vi "OpenLEDStrip.vi"(0 "Digital Module (Module 1)":T2, 1 "Max Duty Cycle (1)":sgl=1.0, 5 "DIO Channel Red":T1, 7 "DIO Channel Green":T1, 9 "DIO Channel Blue":T1, 11 "error in (no error)":errorcluster, 12 "PWM Rate (Hz)":sgl=1000.0) -> (4 "LEDStripRef":T3={"PWM Rate (Hz)"=1000.0, "Max Duty Cycle"=1000.0, "DigitalOutputRed"={"Digital Module"=enum."Digital Module 1", "DIO Channel"=enum."DIO 1", "DevStatus"={"status"=FALSE, "code"=0, "source"=""}}, "DigitalOutputGreen"={"Digital Module"=enum."Digital Module 1", "DIO Channel"=enum."DIO 1", "DevStatus"={"status"=FALSE, "code"=0, "source"=""}}, "DigitalOutputBlue"={"Digital Module"=enum."Digital Module 1", "DIO Channel"=enum."DIO 1", "DevStatus"={"status"=FALSE, "code"=0, "source"=""}}, "DevStatus"={"status"=FALSE, "code"=0, "source"=""}}, 15 "error out":errorcluster)   [LabVIEW 2013]
uses:
  LEDStripRef.ctl
  <vilib>/Rock Robotics/WPI/DigitalOutput/WPI_DigitalOutputDevRef.ctl
  <vilib>/Rock Robotics/SystemInterfaces/Typedef/FPGA_TypedefDigitalModule.ctl
  <vilib>/Rock Robotics/SystemInterfaces/DIO/FPGA_DIOChannel.ctl
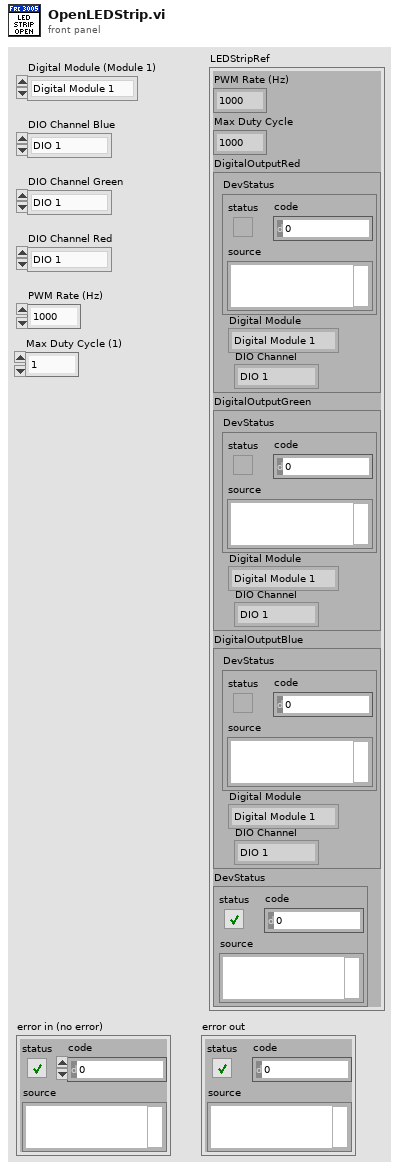
[diagram p1: front panel]
types:
  T1 = typedef "FPGA_DIOChannel.ctl" = enum8{"DIO 1", "DIO 2", "DIO 3", "DIO 4", "DIO 5", "DIO 6", "DIO 7", "DIO 8", "DIO 9", "DIO 10", "DIO 11", "DIO 12", "DIO 13", "DIO 14", "Invalid"}
  T2 = typedef "FPGA_TypedefDigitalModule.ctl" = enum16{"Digital Module 1", "Digital Module 2"}
  T3 = typedef "LEDStripRef.ctl" = cluster{"PWM Rate (Hz)":sgl, "Max Duty Cycle":sgl, "DigitalOutputRed":T4, "DigitalOutputGreen":T4, "DigitalOutputBlue":T4, "DevStatus":errorcluster}
  T4 = typedef "WPI_DigitalOutputDevRef.ctl" = cluster{"Digital Module":T2, "DIO Channel":T1, "DevStatus":errorcluster}
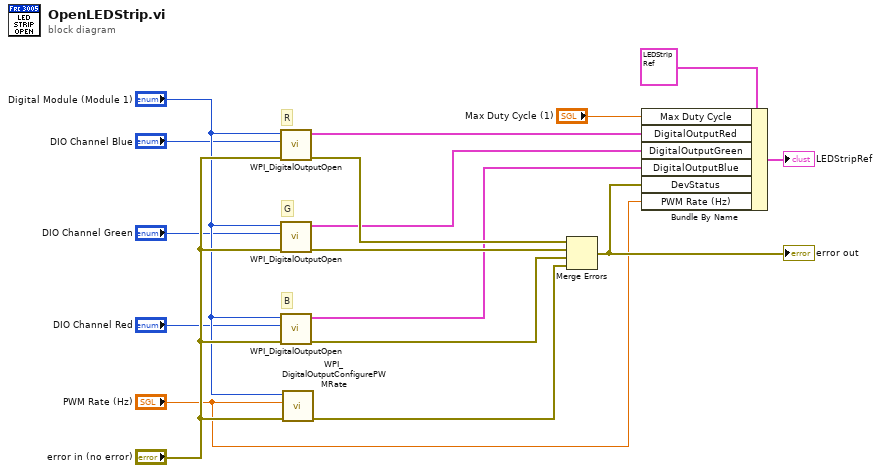
[diagram p0: block diagram]
diagram:
  # "B"
  # "G"
  # "R"
  n1 = call <vilib>:"WPI_DigitalOutputOpen.vi"("error in (no error)"="error in (no error)", "DIO Channel"="DIO Channel Blue", "Digital Module (Module 1)"="Digital Module (Module 1)") -> ("error out"=w10:errorcluster, "DigitalOutputDevRef"=w6:T4)  [unwired: 7 in]
  n2 = call <vilib>:"WPI_DigitalOutputOpen.vi"("error in (no error)"="error in (no error)", "DIO Channel"="DIO Channel Green", "Digital Module (Module 1)"="Digital Module (Module 1)") -> ("error out"=w11:errorcluster, "DigitalOutputDevRef"=w5:T4)  [unwired: 7 in]
  n3 = call <vilib>:"WPI_DigitalOutputOpen.vi"("error in (no error)"="error in (no error)", "DIO Channel"="DIO Channel Red", "Digital Module (Module 1)"="Digital Module (Module 1)") -> ("error out"=w12:errorcluster, "DigitalOutputDevRef"=w4:T4)  [unwired: 7 in]
  n4 = call <vilib>:"WPI_DigitalOutputConfigurePWMRate.vi"("error in (no error)"="error in (no error)", "PWM Rate (Hz)"="PWM Rate (Hz)", "DIO Module"="Digital Module (Module 1)") -> ("error out"=w15:errorcluster)  [unwired: 8 in]
  n5 = Merge Errors(w10, w11, w12, w15) -> (w3:errorcluster)
  "error out" <- w3
  n6 = Bundle By Name(cluster=T3 {"PWM Rate (Hz)"=0.0, "Max Duty Cycle"=0.0, "DigitalOutputRed"={"Digital Module"=enum."Digital Module 1", "DIO Channel"=enum."DIO 1", "DevStatus"={"status"=FALSE, "code"=0, "source"=""}}, "DigitalOutputGreen"={"Digital Module"=enum."Digital Module 1", "DIO Channel"=enum."DIO 1", "DevStatus"={"status"=FALSE, "code"=0, "source"=""}}, "DigitalOutputBlue"={"Digital Module"=enum."Digital Module 1", "DIO Channel"=enum."DIO 1", "DevStatus"={"status"=FALSE, "code"=0, "source"=""}}, "DevStatus"={"status"=FALSE, "code"=0, "source"=""}} ("LEDStripRef"), "Max Duty Cycle"="Max Duty Cycle (1)", "DigitalOutputRed"=w6, "DigitalOutputGreen"=w5, "DigitalOutputBlue"=w4, "DevStatus"=w3, "PWM Rate (Hz)"="PWM Rate (Hz)") -> (→"LEDStripRef":T3)
